vi "TextBoxCtrlMgr.Append Text.vi"(7 "Text In":string, 10 "error in (no error)":errorcluster, 11 "TextBoxLogCtrlMgr in":refnum<class "TextBoxLogCtrlMgr.lvclass">) -> (2 "error out":errorcluster, 3 "TextBoxLogCtrlMgr out":refnum<class "TextBoxLogCtrlMgr.lvclass">)   [LabVIEW 2017, in "TextBoxLogCtrlMgr.lvclass"]
uses:
  TextBoxLogCtrlMgr.lvclass
  TextBoxLogCtrlMgr.lvclass/TextBoxLogCtrlMgr.ctl
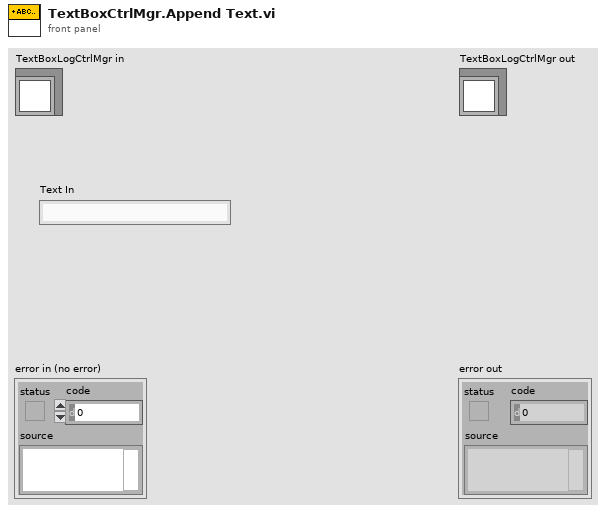
[diagram p1: front panel]
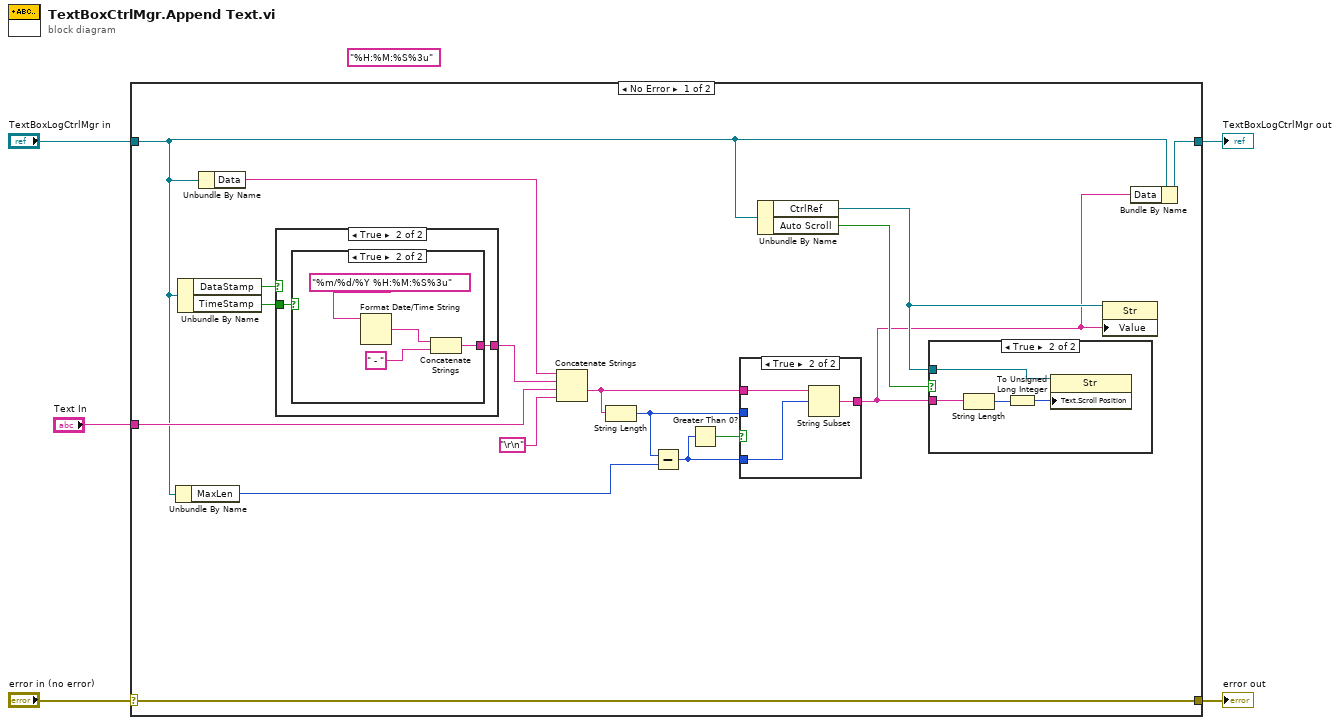
[diagram p0: block diagram]
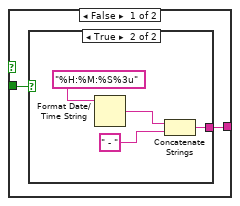
[diagram p2: hidden frame]
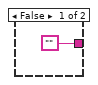
[diagram p3: hidden frame]
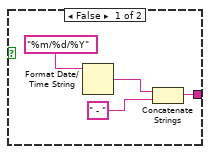
[diagram p4: hidden frame]
diagram:
  (unwired) "%H:%M:%S%3u" ("time format string (%c)")
  n1 = case shown="No Error" "error in (no error)" {
    selector: "error in (no error)" -> [w22 w49]
    tunnel: [w22 w49] -> w4
    tunnel: [w21 w48] -> w2
    tunnel: "TextBoxLogCtrlMgr in" -> [w8 w48]
    tunnel: "Text In" -> [w9 _]
    frame No Error {
      n2 = Unbundle By Name(w8) -> ("MaxLen"=w17:i32)
      n3 = Unbundle By Name(w8) -> ("DataStamp"=w7:bool, "TimeStamp"=w6:bool)
      n4 = Unbundle By Name(w8) -> ("Data"=w11:string)
      n5 = case shown="True" w7 {
        tunnel: [w23 w31] -> w10
        tunnel: w6 -> [w24 w30]
        frame False {
          n6 = case shown="True" w24 {
            tunnel: ["" w26] -> w23
            frame False {
            }
            frame True {
              n7 = Format Date/Time String(time format string (%c)="%H:%M:%S%3u") -> (date/time string=w29:string)  [unwired: 2 in]
              n8 = Concatenate Strings(w29, " - ") -> (w26:string)
            }
          }
        }
        frame True {
          n9 = case shown="True" w30 {
            tunnel: [w33 w36] -> w31
            frame False {
              n10 = Format Date/Time String(time format string (%c)="%m/%d/%Y") -> (date/time string=w35:string)  [unwired: 2 in]
              n11 = Concatenate Strings(w35, " - ") -> (w33:string)
            }
            frame True {
              n12 = Format Date/Time String(time format string (%c)="%m/%d/%Y %H:%M:%S%3u") -> (date/time string=w39:string)  [unwired: 2 in]
              n13 = Concatenate Strings(w39, " - ") -> (w36:string)
            }
          }
        }
      }
      n14 = Concatenate Strings(w11, w10, w9, "\r\n") -> (w13:string)
      n15 = String Length(string=w13) -> (length=w19:i32)
      n16 = Subtract(x=w19, y=w17) -> (x-y=w18:i32)
      n17 = Greater Than 0?(x=w18) -> (x > 0?=w20:bool)
      n18 = case shown="True" w20 {
        tunnel: w19 -> [_ _]
        tunnel: w18 -> [_ w46]
        tunnel: w13 -> [w44 w47]
        tunnel: [w44 w45] -> w14
        frame False {
        }
        frame True {
          n19 = String Subset(string=w47, offset (0)=w46) -> (substring=w45:string)  [unwired: 1 in]
        }
      }
      n20 = Unbundle By Name(w8) -> ("CtrlRef"=w15:refnum<vi>, "Auto Scroll"=w16:bool)
      n21 = case shown="True" w16 {
        tunnel: w14 -> [_ w43]
        tunnel: w15 -> [_ w42]
        frame False {
        }
        frame True {
          n22 = String Length(string=w43) -> (length=w41:i32)
          n23 = To Unsigned Long Integer(number=w41) -> (unsigned 32bit integer=w40:u32)
          n24 = property class="Str"(reference=w42, "Text.Scroll Position"=w40) -> ()  [unwired: 1 in, 2 out]
        }
      }
      n25 = property class="Str"(reference=w15, "Value"=w14) -> ()  [unwired: 1 in, 2 out]
      n26 = Bundle By Name(cluster=w8, "Data"=w14) -> (w21:refnum<class "TextBoxLogCtrlMgr.lvclass">)
    }
    frame Error {
    }
  }
  "error out" <- w4
  "TextBoxLogCtrlMgr out" <- w2
